vi "read config.vi"(8 "error in (no error)":errorcluster, 9 "data value reference":refnum<data-value>, 10 "file path (use dialog)":path, 11 "hardware in":refnum<class "hardware.lvclass">) -> (0 "error out":errorcluster, 3 "hardware out":refnum<class "hardware.lvclass">)   [LabVIEW 2025, in "hardware.lvclass"]
uses:
  hardware.lvclass
  hardware.lvclass/hardware.ctl
  264ae7df-eee7-4ea2-a5dd-e1c985cff494.vi
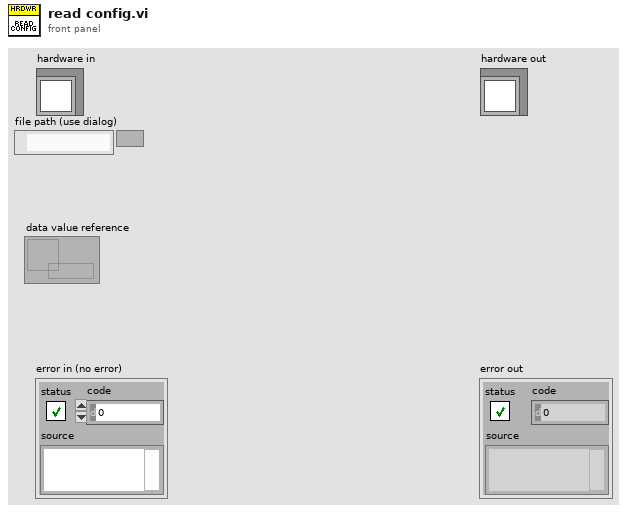
[diagram p1: front panel]
types:
  T1 = cluster{"TC_Port":string, "Relay_Port":string, "Relay_Values":refnum<data-value>}
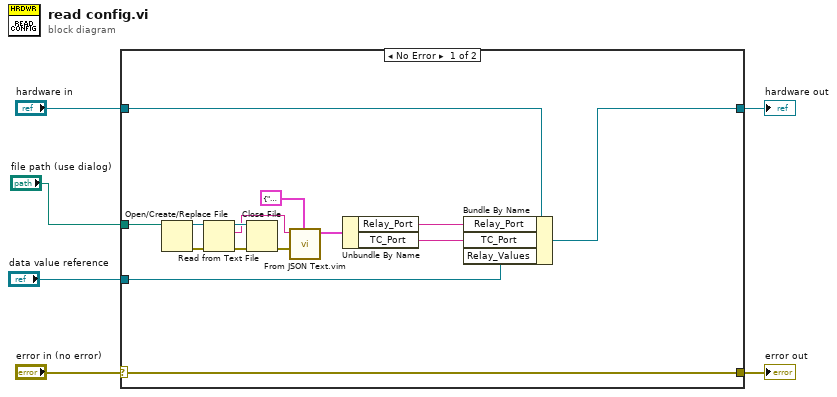
[diagram p0: block diagram]
diagram:
  n1 = case shown="No Error" "error in (no error)" {
    selector: "error in (no error)" -> [w21 w23]
    tunnel: [w21 w23] -> w5
    tunnel: [w7 w22] -> w3
    tunnel: "hardware in" -> [w11 w22]
    tunnel: "file path (use dialog)" -> [w13 _]
    tunnel: "data value reference" -> [w8 _]
    frame No Error {
      n2 = Open/Create/Replace File(file path (use dialog)=w13) -> (refnum out=w17:refnum<file>, error out=w20:errorcluster)  [unwired: 5 in, 1 out]
      n3 = Read from Text File(file (use dialog)=w17, error in=w20) -> (refnum out=w18:refnum<file>, text=w16:string, error out=w19:errorcluster)  [unwired: 2 in, 1 out]
      n4 = Close File(refnum=w18, error in=w19) -> (error out=w15:errorcluster)  [unwired: 1 out]
      n5 = call "From JSON Text.vim"("Data Type and Default Value"=T1 {"TC_Port"="", "Relay_Port"="", "Relay_Values"=refnum}, "error in (no error)"=w15, "JSON"=w16) -> ("Data out"=w12:T1)  [unwired: 7 in, 1 out]
      n6 = Unbundle By Name(w12) -> ("Relay_Port"=w10:string, "TC_Port"=w9:string)
      n7 = Bundle By Name(cluster=w11, "Relay_Port"=w10, "TC_Port"=w9, "Relay_Values"=w8) -> (w7:refnum<class "hardware.lvclass">)
    }
    frame Error {
    }
  }
  "error out" <- w5
  "hardware out" <- w3
